vi "RSZVB Set Reference Discrete Marker.vi"(7 "Mode (0)":i32(ring) items=["Continuous", "Discrete"], 8 "error in (no error)":errorcluster {"code" format="%.0x"}, 9 "Marker (1)":i32=1, 10 "Channel (Trace) (1)":i32=1, 11 "VISA session":refnum<visa-resource-name>) -> (0 "error out":errorcluster {"code" format="%.0x"}, 3 "dup VISA session":refnum<visa-resource-name>)   [LabVIEW 2011]
doc: "Sets the reference marker to continuous or discrete mode. The marker doesn't have to be created before (CALCulate<Chn>:MARKer<Mk>:REFerence[:STATe] ON), the mode can be assigned in advance. \n\n\nRemote-control command(s):\nCALCulate<Chn>:MARKer<Mk>:REFerence:MODE CONTinuous | DISCrete"
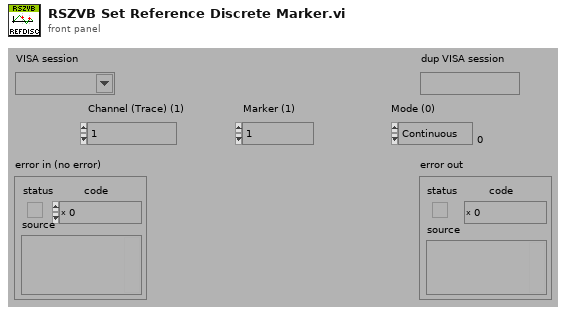
[diagram p1: front panel]
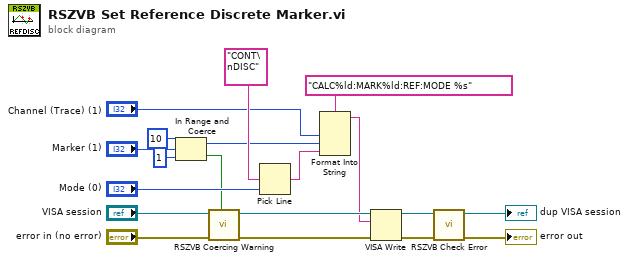
[diagram p0: block diagram]
diagram:
  n1 = In Range and Coerce(upper limit=10, x="Marker (1)", lower limit=1) -> (coerced(x)=w9:i32, In Range?=w12:bool)
  n2 = call "RSZVB Coercing Warning.vi"("In Range?"=w12, "error in (no error)"="error in (no error)", "VISA session"="VISA session") -> ("error out"=w7:errorcluster, "dup VISA session"=w6:refnum<visa-resource-name>)  [unwired: 7 in]
  n3 = Pick Line(multi-line string="CONT\nDISC", line index="Mode (0)") -> (output string=w8:string)  [unwired: 1 in]
  n4 = Format Into String(format string="CALC%ld:MARK%ld:REF:MODE %s", "Channel (Trace) (1)", w9, w8) -> (resulting string=w5:string)  [unwired: 2 in, 1 out]
  n5 = VISA Write(VISA resource name=w6, write buffer=w5, error in (no error)=w7) -> (VISA resource name out=w3:refnum<visa-resource-name>, error out=w4:errorcluster)  [unwired: 1 out]
  n6 = call "RSZVB Check Error.vi"("error in (no error)"=w4, "VISA session"=w3) -> ("error out"=→"error out":errorcluster, "dup VISA session"=→"dup VISA session":refnum<visa-resource-name>)  [unwired: 8 in]
